vi "WriteDataFile.vi"(9 "数据输入":cluster{"数组":dbl[]}[](array[cluster]), 10 "首行":string[](array[string]), 11 "保存路径":path) -> ()   [LabVIEW 2018, in "DataDisplay.lvlib"]
uses:
  DataDisplay.lvlib
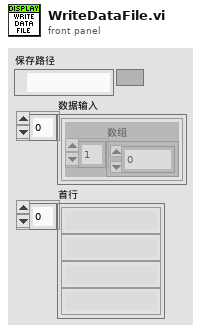
[diagram p1: front panel]
types:
  T1 = enum16{"open", "replace", "create", "open or create", "replace or create", "replace or create with confirmation"}
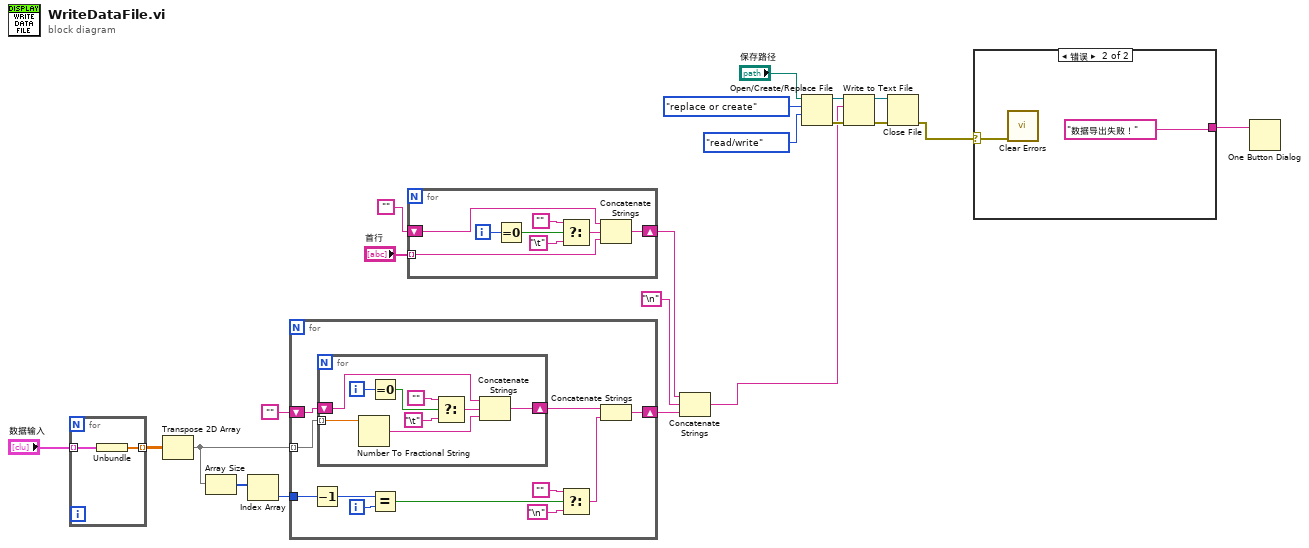
[diagram p0: block diagram]
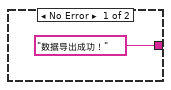
[diagram p2: hidden frame]
diagram:
  n1 = for {
    tunnel: "数据输入" -> [w23] mode=indexing
    tunnel: [w22] -> w20 mode=indexing
    n2 = Unbundle(w23) -> ("数组"=w22:dbl[])
  }
  n3 = Transpose 2D Array(2D array=w20) -> (transposed array=w18:dbl[][])
  n4 = Array Size(array=w18) -> (size(s)=w17:i32[])
  n5 = Index Array(array=w17) -> (element=w16:i32)  [unwired: 1 in]
  n6 = for {
    tunnel: w18 -> [w34] mode=indexing
    shift-right: [w25] -> w11
    shift-left: "" -> [w33]
    tunnel: w16 -> [w30]
    i -> [w31]
    n7 = Decrement(x=w30) -> (x-1=w29:i32)
    n8 = for {
      tunnel: w34 -> [w43] mode=indexing
      shift-right: [w37] -> w32
      shift-left: w33 -> [w42]
      i -> [w41]
      n9 = Number To Fractional String(number=w43) -> (F-format string=w35:string)  [unwired: 3 in]
      n10 = Equal To 0?(x=w41) -> (x = 0?=w40:bool)
      n11 = Select(t="", s=w40, f="\t") -> (s? t:f=w36:string)
      n12 = Concatenate Strings(w42, w36, w35) -> (w37:string)
    }
    n13 = Equal?(x=w29, y=w31) -> (x = y?=w28:bool)
    n14 = Select(t="", s=w28, f="\n") -> (s? t:f=w24:string)
    n15 = Concatenate Strings(w32, w24) -> (w25:string)
  }
  n16 = for {
    shift-right: [w46] -> w13
    shift-left: "" -> [w51]
    tunnel: "首行" -> [w44] mode=indexing
    i -> [w50]
    n17 = Equal To 0?(x=w50) -> (x = 0?=w49:bool)
    n18 = Select(t="", s=w49, f="\t") -> (s? t:f=w45:string)
    n19 = Concatenate Strings(w51, w45, w44) -> (w46:string)
  }
  n20 = Concatenate Strings(w13, "\n", w11) -> (w5:string)
  n21 = Open/Create/Replace File(file path (use dialog)="保存路径", operation (0:open)=T1."replace or create" ("操作(0:open)"), access (0:read/write)=enum16{"read/write", "read-only", "write-only"}."read/write" ("权限(0:read/write)")) -> (refnum out=w7:refnum<file>, error out=w6:errorcluster)  [unwired: 3 in, 1 out]
  n22 = Write to Text File(file (use dialog)=w7, text=w5, error in=w6) -> (refnum out=w3:refnum<file>, error out=w4:errorcluster)  [unwired: 1 in, 1 out]
  n23 = Close File(refnum=w3, error in=w4) -> (error out=w2:errorcluster)  [unwired: 1 out]
  n24 = case shown="错误" w2 {
    selector: w2 -> [_ w53]
    tunnel: ["数据导出成功！" "数据导出失败！"] -> w1
    frame No Error {
    }
    frame Error {
      n25 = call <vilib>:"Clear Errors.vi"("error in (no error)"=w53) -> ()  [unwired: 5 in, 2 out]
    }
  }
  n26 = One Button Dialog(message=w1) -> ()  [unwired: 1 in, 1 out]
